vi "Write_to_TDMS.vi"(8 "error in (no error)":errorcluster, 9 "Array":bool[](array[boolean]), 10 "output cluster":T1, 11 "Refnum in":refnum<k34>) -> (3 "Refnum out":refnum<k34>)   [LabVIEW 2021]
panel:
  out "Array 4":dbl[][](array[numeric])
  out "Array 3":dbl[][](array[numeric])
  out "Array 2":dbl[][](array[numeric])
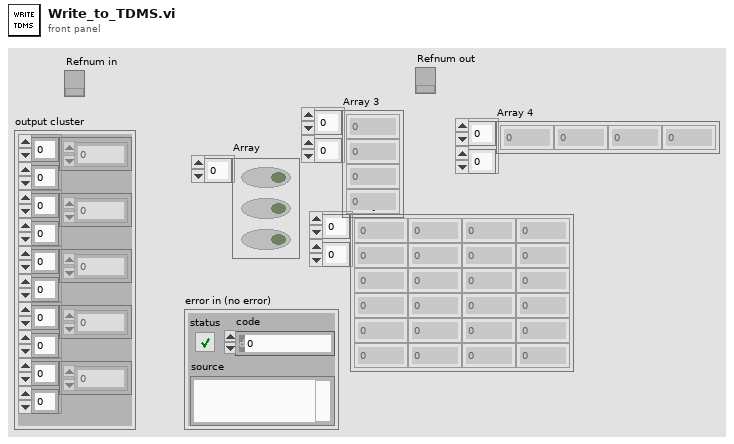
[diagram p1: front panel]
types:
  T1 = cluster{dbl[][], dbl[][], dbl[][], dbl[][], dbl[][]}
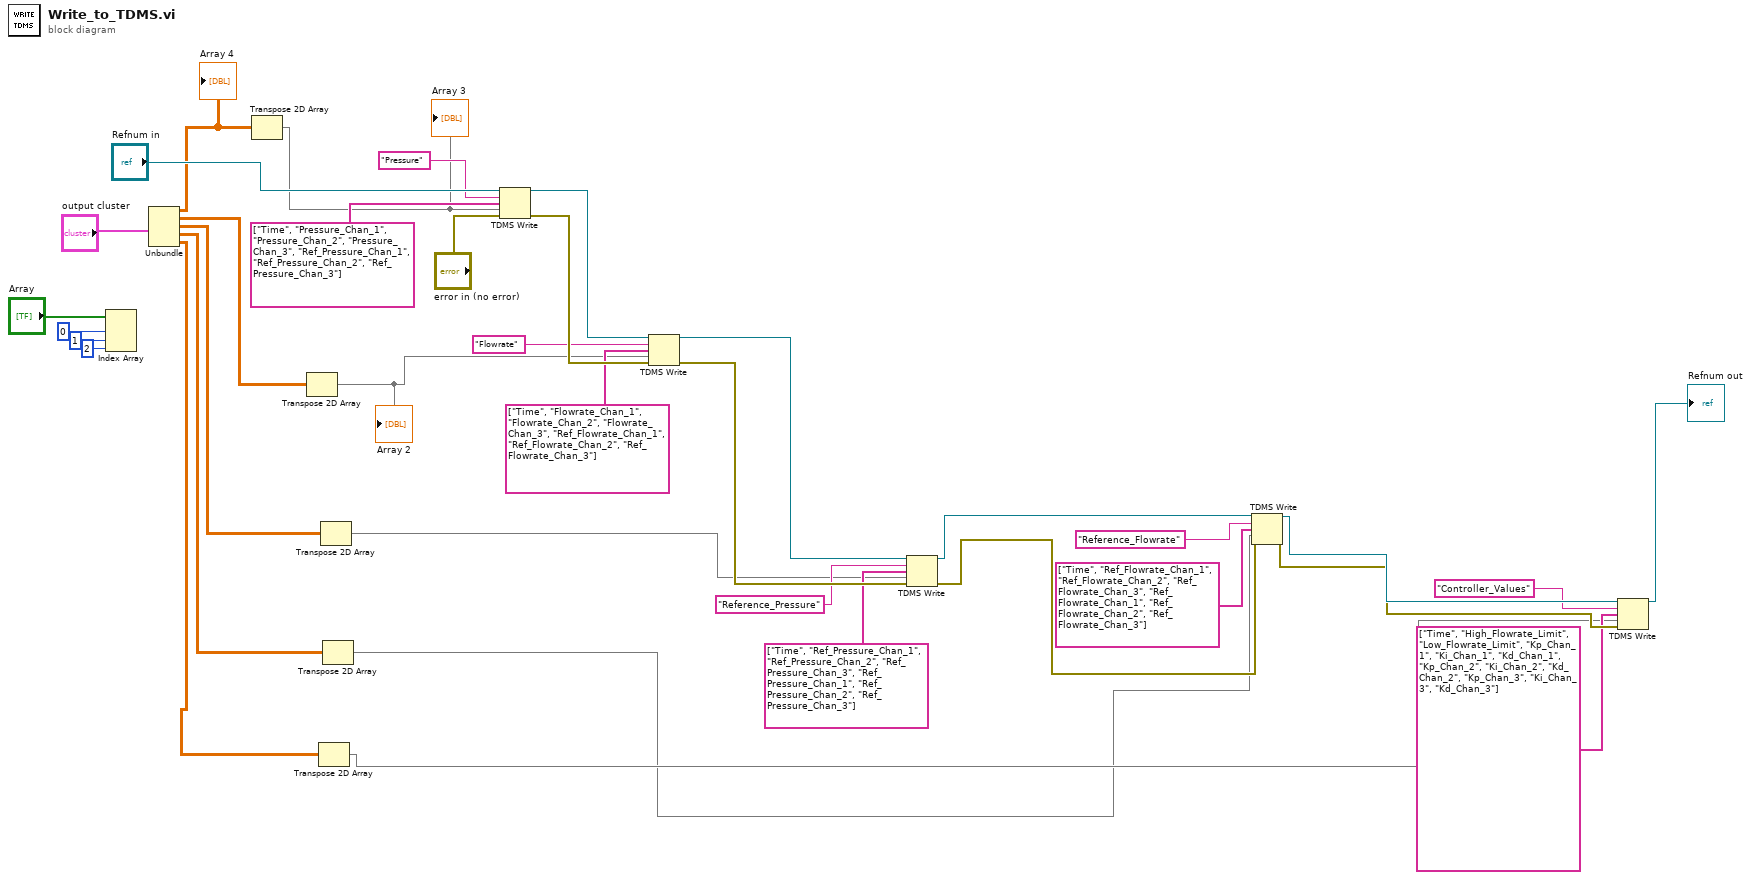
[diagram p0: block diagram]
diagram:
  n1 = Index Array(array="Array", index #1=0 ("index"), index #2=1 ("index"), index #3=2 ("index")) -> ()  [unwired: 3 out]
  n2 = Unbundle("output cluster") -> (w10:dbl[][], w2:dbl[][], w4:dbl[][], w6:dbl[][], w8:dbl[][])
  "Array 4" <- w10
  n3 = Transpose 2D Array(2D array=w10) -> (transposed array=w9:dbl[][])
  "Array 3" <- w9
  n4 = Transpose 2D Array(2D array=w2) -> (transposed array=w1:dbl[][])
  "Array 2" <- w1
  n5 = Transpose 2D Array(2D array=w8) -> (transposed array=w7:dbl[][])
  n6 = Transpose 2D Array(2D array=w4) -> (transposed array=w3:dbl[][])
  n7 = Transpose 2D Array(2D array=w6) -> (transposed array=w5:dbl[][])
  n8 = TDMS Write(0:"Refnum in", 5:"Pressure" ("group name in (Untitled)"), 7:string[] ["Time", "Pressure_Chan_1", "Pressure_Chan_2", "Pressure_Chan_3", "Ref_Pressure_Chan_1", "Ref_Pressure_Chan_2", "Ref_Pressure_Chan_3"] ("channel name(s) in (Untitled)"), 9:w9, 11:"error in (no error)") -> (4:w31:refnum<k34>, 15:w30:errorcluster)  [unwired: 1 in, 2 out]
  n9 = TDMS Write(0:w31, 5:"Flowrate" ("group name in (Untitled)"), 7:string[] ["Time", "Flowrate_Chan_1", "Flowrate_Chan_2", "Flowrate_Chan_3", "Ref_Flowrate_Chan_1", "Ref_Flowrate_Chan_2", "Ref_Flowrate_Chan_3"] ("channel name(s) in (Untitled)"), 9:w1, 11:w30) -> (4:w26:refnum<k34>, 15:w27:errorcluster)  [unwired: 1 in, 2 out]
  n10 = TDMS Write(0:w26, 5:"Reference_Pressure" ("group name in (Untitled)"), 7:string[] ["Time", "Ref_Pressure_Chan_1", "Ref_Pressure_Chan_2", "Ref_Pressure_Chan_3", "Ref_Pressure_Chan_1", "Ref_Pressure_Chan_2", "Ref_Pressure_Chan_3"] ("channel name(s) in (Untitled)"), 9:w3, 11:w27) -> (4:w25:refnum<k34>, 15:w22:errorcluster)  [unwired: 1 in, 2 out]
  n11 = TDMS Write(0:w25, 5:"Reference_Flowrate" ("group name in (Untitled)"), 7:string[] ["Time", "Ref_Flowrate_Chan_1", "Ref_Flowrate_Chan_2", "Ref_Flowrate_Chan_3", "Ref_Flowrate_Chan_1", "Ref_Flowrate_Chan_2", "Ref_Flowrate_Chan_3"] ("channel name(s) in (Untitled)"), 9:w5, 11:w22) -> (4:w24:refnum<k34>, 15:w21:errorcluster)  [unwired: 1 in, 2 out]
  n12 = TDMS Write(0:w24, 5:"Controller_Values" ("group name in (Untitled)"), 7:string[] ["Time", "High_Flowrate_Limit", "Low_Flowrate_Limit", "Kp_Chan_1", "Ki_Chan_1", "Kd_Chan_1", "Kp_Chan_2", "Ki_Chan_2", "Kd_Chan_2", "Kp_Chan_3", "Ki_Chan_3", "Kd_Chan_3"] ("channel name(s) in (Untitled)"), 9:w7, 11:w21) -> (4:→"Refnum out":refnum<k34>)  [unwired: 1 in, 3 out]
